vi "Hc2SequenceRunner.vi"() -> ()   [LabVIEW 2019]
uses:
  Components/DeltaRamp_globals.vi
  Components/B_Globals.vi
  Components/Global 2.vi
panel:
  in  "Set":bool
  in  "App":bool
  out "Settle Progress":u8(slide)=98 scale=0.0..100.0
  in  "Settle [Min]":dbl=1.0
  out "Numeric":i32=7
  in  "Base Name":string="RT_100uA"
  in  "Start":bool
  in  "Directory":path=path "C:/User Data/gy251/20210625 karine1B_Nb40-Dy20-Nb20-MgO2-Nb30/Out-of-plane"
  in  "T_high [K]":dbl=10.0
  in  "T_low [K]":dbl=2.0
  in  "dT/dt [K/min]":dbl=0.3
  in  "B_rate [T/min]":dbl=0.2
  in  "Set Fields, T_low, T_high":dbl[][](array[numeric])=[[0.0, 2.0, 10.0], [0.2, 2.0, 10.0], [0.4, 2.0, 10.0], [0.6, 2.0, 10.0], [0.8, 2.0, 10.0], [1.0, 2.0, 10.0], [1.5, 2.0, 10.0], [2.0, 2.0, 10.0], [2.5, 2.0, 10.0], [3.0, 2.0, 10.0], [3.5, 2.0, 10.0]]
  out "Action":string="Done/Wait for Start"
  out "Output File":path=path "RT_100uAapp=2p00T"
  # "Defaults"
  # "T_high -> Apply Field -> T_low"
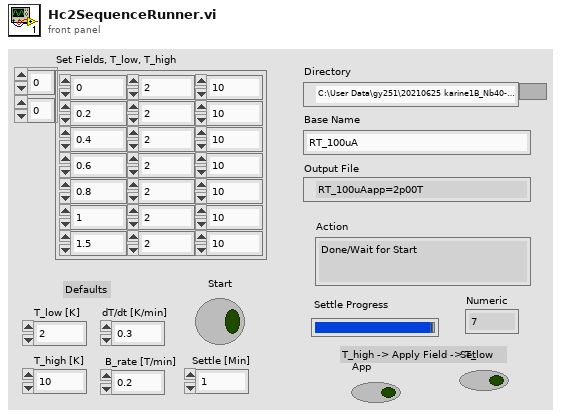
[diagram p1: front panel]
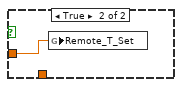
[diagram p3: hidden frame]
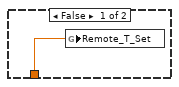
[diagram p4: hidden frame]
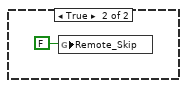
[diagram p5: hidden frame]
diagram:
  w2 = path ""
  n1 = global write "DeltaRamp_globals.vi" "Remote_Save_Directory"(w2) -> ()
  n2 = global write "DeltaRamp_globals.vi" "Remote_Ramp_Path"(w2) -> ()
  n3 = global write "DeltaRamp_globals.vi" "Remote_Save_String"("") -> ()
  n4 = while {
    stop <- FALSE stop-if-true
    n5 = local write "Action"("Done/Wait for Start") -> ()
    n6 = case shown="True" "Start" {
      frame False {
      }
      frame True {
        n7 = for {
          tunnel: "Set Fields, T_low, T_high" -> [w104] mode=indexing
          tunnel: "B_rate [T/min]" -> [w103]
          tunnel: "Directory" -> [w102]
          tunnel: "Base Name" -> [w101]
          tunnel: "T_low [K]" -> [w100]
          tunnel: "dT/dt [K/min]" -> [w99]
          tunnel: "T_high [K]" -> [w66]
          i -> [w98]
          n8 = flat-sequence {
            tunnel: w104 -> [w120]
            tunnel: w103 -> [w136]
            tunnel: w101 -> [w134]
            tunnel: [w127] -> w83
            tunnel: [w135] -> w81
            tunnel: w102 -> [w135]
            tunnel: [w122] -> w79
            tunnel: [w119] -> w77
            tunnel: w83 -> [w141]
            tunnel: [w141] -> w82
            tunnel: w81 -> [w140]
            tunnel: [w140] -> w80
            tunnel: w79 -> [w139]
            tunnel: [w139] -> w78
            tunnel: w77 -> [w138]
            tunnel: [w138] -> w76
            tunnel: [w143] -> w118
            tunnel: w82 -> [w143]
            tunnel: w80 -> [w142]
            tunnel: [w142] -> w117
            tunnel: w78 -> [w144]
            tunnel: w76 -> [w145]
            tunnel: [w145] -> w93
            tunnel: [w144] -> w88
            tunnel: w118 -> [w149]
            tunnel: [w149] -> w116
            tunnel: w117 -> [w148]
            tunnel: [w148] -> w115
            tunnel: [w147] -> w94
            tunnel: w93 -> [w147]
            tunnel: [w146] -> w89
            tunnel: w88 -> [w146]
            tunnel: [w153] -> w114
            tunnel: w116 -> [w153]
            tunnel: [w152] -> w113
            tunnel: w115 -> [w152]
            tunnel: [w151] -> w95
            tunnel: w94 -> [w151]
            tunnel: [w150] -> w90
            tunnel: w89 -> [w150]
            tunnel: [w162] -> w65
            tunnel: w114 -> [w162]
            tunnel: [w161] -> w63
            tunnel: w113 -> [w161]
            tunnel: [w160] -> w61
            tunnel: w95 -> [w160]
            tunnel: [w157] -> w59
            tunnel: w90 -> [w157]
            tunnel: w66 -> [w159]
            tunnel: w65 -> [w169]
            tunnel: [w169] -> w64
            tunnel: w63 -> [w168]
            tunnel: [w168] -> w62
            tunnel: w61 -> [w167]
            tunnel: [w167] -> w60
            tunnel: w59 -> [w166]
            tunnel: [w166] -> w58
            tunnel: [w174] -> w57
            tunnel: w64 -> [w174]
            tunnel: [w173] -> w55
            tunnel: w62 -> [w173]
            tunnel: [w172] -> w53
            tunnel: w60 -> [w172]
            tunnel: [w171] -> w51
            tunnel: w58 -> [w171]
            tunnel: w57 -> [w178]
            tunnel: [w178] -> w56
            tunnel: w55 -> [w177]
            tunnel: [w177] -> w54
            tunnel: w53 -> [w176]
            tunnel: [w176] -> w52
            tunnel: w51 -> [w175]
            tunnel: [w175] -> w50
            tunnel: [w184] -> w112
            tunnel: w56 -> [w184]
            tunnel: [w183] -> w111
            tunnel: w54 -> [w183]
            tunnel: [w182] -> w96
            tunnel: w52 -> [w182]
            tunnel: [w181] -> w91
            tunnel: w50 -> [w181]
            tunnel: w112 -> [w189]
            tunnel: w111 -> [w190]
            tunnel: [w190] -> w110
            tunnel: [w189] -> w109
            tunnel: [w188] -> w97
            tunnel: w96 -> [w188]
            tunnel: [w187] -> w92
            tunnel: w91 -> [w187]
            tunnel: [w198] -> w43
            tunnel: w110 -> [w198]
            tunnel: [w197] -> w41
            tunnel: w109 -> [w197]
            tunnel: [w196] -> w39
            tunnel: w97 -> [w196]
            tunnel: [w195] -> w37
            tunnel: w92 -> [w195]
            tunnel: w43 -> [w209]
            tunnel: [w209] -> w42
            tunnel: w41 -> [w207]
            tunnel: [w207] -> w40
            tunnel: w39 -> [w214]
            tunnel: [w214] -> w38
            tunnel: w37 -> [w213]
            tunnel: [w213] -> w36
            tunnel: [w218] -> w108
            tunnel: w42 -> [w218]
            tunnel: [w217] -> w107
            tunnel: w40 -> [w217]
            tunnel: w38 -> [w216]
            tunnel: w36 -> [w215]
            tunnel: [w216] -> w87
            tunnel: [w215] -> w84
            tunnel: w100 -> [w224]
            tunnel: w108 -> [w223]
            tunnel: w107 -> [w228]
            tunnel: [w228] -> w49
            tunnel: w99 -> [w221]
            tunnel: w87 -> [w222]
            tunnel: [w227] -> w47
            tunnel: w84 -> [w227]
            tunnel: [w223] -> w45
            tunnel: [w222] -> w30
            tunnel: [w221] -> w24
            tunnel: w49 -> [w237]
            tunnel: [w237] -> w48
            tunnel: w47 -> [w236]
            tunnel: [w236] -> w46
            tunnel: w45 -> [w235]
            tunnel: [w235] -> w44
            tunnel: [w233] -> w31
            tunnel: w30 -> [w233]
            tunnel: [w232] -> w25
            tunnel: w24 -> [w232]
            tunnel: [w242] -> w106
            tunnel: w48 -> [w242]
            tunnel: [w241] -> w85
            tunnel: w46 -> [w241]
            tunnel: [w240] -> w74
            tunnel: w44 -> [w240]
            tunnel: [w239] -> w32
            tunnel: w31 -> [w239]
            tunnel: [w238] -> w26
            tunnel: w25 -> [w238]
            tunnel: w106 -> [w249]
            tunnel: [w249] -> w105
            tunnel: [w248] -> w86
            tunnel: w85 -> [w248]
            tunnel: [w247] -> w75
            tunnel: w74 -> [w247]
            tunnel: [w246] -> w67
            tunnel: [w245] -> w33
            tunnel: w32 -> [w245]
            tunnel: [w244] -> w27
            tunnel: w26 -> [w244]
            tunnel: w105 -> [w259]
            tunnel: [w259] -> w73
            tunnel: w86 -> [w258]
            tunnel: [w258] -> w71
            tunnel: [w257] -> w69
            tunnel: w75 -> [w257]
            tunnel: w67 -> [w256]
            tunnel: [w255] -> w34
            tunnel: w33 -> [w255]
            tunnel: [w254] -> w28
            tunnel: w27 -> [w254]
            tunnel: w73 -> [w267]
            tunnel: [w267] -> w72
            tunnel: w71 -> [w266]
            tunnel: [w266] -> w70
            tunnel: w69 -> [w265]
            tunnel: [w265] -> w68
            tunnel: [w263] -> w35
            tunnel: w34 -> [w263]
            tunnel: [w262] -> w29
            tunnel: w28 -> [w262]
            tunnel: w72 -> [w269]
            tunnel: [w272] -> w23
            tunnel: w70 -> [w272]
            tunnel: w68 -> [w268]
            tunnel: w35 -> [w271]
            tunnel: w29 -> [w270]
            tunnel: [w271] -> w21
            tunnel: [w270] -> w19
            tunnel: [w269] -> w17
            tunnel: [w268] -> w15
            tunnel: w23 -> [w278]
            tunnel: [w278] -> w22
            tunnel: w21 -> [w277]
            tunnel: [w277] -> w20
            tunnel: w19 -> [w276]
            tunnel: [w276] -> w18
            tunnel: w17 -> [w275]
            tunnel: [w275] -> w16
            tunnel: w15 -> [w274]
            tunnel: [w274] -> w14
            tunnel: w22 -> [w281]
            tunnel: w66 -> [_]
            tunnel: w20 -> [w280]
            tunnel: w18 -> [w279]
            tunnel: w16 -> [w283]
            tunnel: w14 -> [w282]
            frame #0 {
              n9 = Index Array(array=w120, index=0) -> (element=w124:dbl)
              n10 = Number To Fractional String(number=w124, precision (6)=2) -> (F-format string=w132:string)  [unwired: 2 in]
              n11 = global write "B_Globals.vi" "Remote_set"(w124) -> ()
              n12 = global write "B_Globals.vi" "Remote_Rate"(w136) -> ()
              n13 = Index Array(array=w120, index=2) -> (element=w122:dbl)
              n14 = Index Array(array=w120, index=1) -> (element=w119:dbl)
              n15 = Search and Replace String(input string=w132, search string=".", replace string="p") -> (result string=w129:string)  [unwired: 5 in, 3 out]
              n16 = Concatenate Strings(w134, "app=", w129, "T") -> (w127:string)
            }
            frame #1 {
              w137 = TRUE
              n17 = global write "B_Globals.vi" "Remote_run"(w137) -> ()
              n18 = global write "B_Globals.vi" "Remote_Go"(w137) -> ()
            }
            frame #2 {
              # "Prep First File"
            }
            frame #3 {
            }
            frame #4 {
              n19 = local write "Action"("Waiting for B stable") -> ()
            }
            frame #5 {
              # "T_low"
              # "T_high"
              n20 = Not Equal?(x=0, y=w157) -> (x != y?=w155:bool)
              n21 = case shown="False" w155 {
                tunnel: w157 -> [_ w164]
                tunnel: w159 -> [w163 _]
                frame False {
                  n22 = global write "Global 2.vi" "Remote_T_Set"(w163) -> ()
                }
                frame True {
                  n23 = global write "Global 2.vi" "Remote_T_Set"(w164) -> ()
                }
              }
              n24 = global write "Global 2.vi" "Remote_T_Rate"(0.5) -> ()
            }
            frame #6 {
              n25 = global write "Global 2.vi" "Remote_T_GoTo"(TRUE) -> ()
            }
            frame #7 {
              n26 = Wait (ms)(milliseconds to wait=20000) -> ()  [unwired: 1 out]
            }
            frame #8 {
              n27 = while {
                stop <- w180 stop-if-true
                n28 = global read "Global 2.vi" "Sample_Stab"() -> (w180:bool)
                n29 = Wait (ms)(milliseconds to wait=500) -> ()  [unwired: 1 out]
              }
            }
            frame #9 {
              n30 = while {
                stop <- w185 stop-if-true
                n31 = global read "B_Globals.vi" "Rem_stable_B"() -> (w185:bool)
                n32 = Wait (ms)(milliseconds to wait=500) -> ()  [unwired: 1 out]
              }
            }
            frame #10 {
              n33 = global write "B_Globals.vi" "Remote_run"(FALSE) -> ()
            }
            frame #11 {
              n34 = Multiply(x="Settle [Min]", y=60) -> (x*y=w192:dbl)
              n35 = for {
                N: w192 -> [w200]
                i -> [w199]
                w206 = 1000
                n36 = Multiply(x=w206, y=w199) -> (x*y=w204:i32)
                n37 = Multiply(x=w206, y=w200) -> (x*y=w205:i32)
                n38 = Wait (ms)(milliseconds to wait=w206) -> ()  [unwired: 1 out]
                n39 = Divide(x=w204, y=w205) -> (x/y=w202:dbl)
                n40 = Multiply(x=100, y=w202) -> (x*y=→"Settle Progress":dbl)
              }
            }
            frame #12 {
              n41 = global write "DeltaRamp_globals.vi" "Remote_Save_Directory"(w209) -> ()
              n42 = Concatenate Strings(w207, "_cool.txt") -> (w211:string)
              n43 = Build Path(base path=w209, name or relative path=w211) -> (appended path=w210:path)
              n44 = String To Path(string=w207) -> (path=w208:path)
              n45 = global write "DeltaRamp_globals.vi" "Remote_Ramp_Path"(w210) -> ()
              n46 = local write "Output File"(w208) -> ()
              n47 = global write "DeltaRamp_globals.vi" "Remote_Save_String"(w211) -> ()
            }
            frame #13 {
              w220 = TRUE
              n48 = global write "DeltaRamp_globals.vi" "Remote_Measure"(w220) -> ()
              n49 = local write "Action"("Starting Measurement") -> ()
              n50 = global write "DeltaRamp_globals.vi" "Remote_Reset"(w220) -> ()
            }
            frame #14 {
              n51 = global write "Global 2.vi" "Remote_T_Rate"(w221) -> ()
              n52 = Not Equal?(x=0, y=w222) -> (x != y?=w226:bool)
              n53 = global write "Global 2.vi" "Remote_T_Ramp"(FALSE) -> ()
              n54 = case shown="True" w226 {
                tunnel: w222 -> [_ w231]
                tunnel: w224 -> [w230 _]
                frame False {
                  n55 = global write "Global 2.vi" "Remote_T_Set"(w230) -> ()
                }
                frame True {
                  n56 = global write "Global 2.vi" "Remote_T_Set"(w231) -> ()
                }
              }
            }
            frame #15 {
              w234 = TRUE
              n57 = global write "Global 2.vi" "Remote_T_Run"(w234) -> ()
              n58 = global write "Global 2.vi" "Remote_T_GoTo"(w234) -> ()
            }
            frame #16 {
              n59 = Wait (ms)(milliseconds to wait=20000) -> ()  [unwired: 1 out]
            }
            frame #17 {
              n60 = while {
                tunnel: [w250] -> w246
                stop <- w251 stop-if-true
                n61 = global read "Global 2.vi" "Sample_Stab"() -> (w252:bool)
                n62 = Wait (ms)(milliseconds to wait=500) -> ()  [unwired: 1 out]
                n63 = global read "DeltaRamp_globals.vi" "Remote_Skip"() -> (w250:bool)
                n64 = Or(x=w250, y=w252) -> (x .or. y?=w251:bool)
              }
            }
            frame #18 {
              n65 = case shown="False" w256 {
                frame False {
                  n66 = global write "DeltaRamp_globals.vi" "Remote_Ramp_Save"(TRUE) -> ()
                }
                frame True {
                  n67 = global write "DeltaRamp_globals.vi" "Remote_Skip"(FALSE) -> ()
                }
              }
            }
            frame #19 {
              n68 = Wait (ms)(milliseconds to wait=1000) -> ()  [unwired: 1 out]
            }
            frame #20 {
            }
            frame #21 {
              n69 = Wait (ms)(milliseconds to wait=1000) -> ()  [unwired: 1 out]
            }
            frame #22 {
              n70 = case shown="True" "Set" {
                tunnel: w280 -> [_ w291]
                tunnel: w279 -> [_ w290]
                tunnel: w283 -> [_ w288]
                tunnel: w282 -> [_ w289]
                tunnel: w281 -> [_ _]
                tunnel: w281 -> [_ w287]
                tunnel: w280 -> [_ w286]
                tunnel: w279 -> [_ w285]
                frame False {
                }
                frame True {
                  n71 = flat-sequence {
                    tunnel: w291 -> [_]
                    tunnel: w290 -> [_]
                    tunnel: w287 -> [w297]
                    tunnel: w289 -> [w304]
                    tunnel: w288 -> [w305]
                    tunnel: w286 -> [w310]
                    tunnel: w285 -> [w309]
                    frame #0 {
                      n72 = global write "B_Globals.vi" "Remote_set"(0.0) -> ()
                    }
                    frame #1 {
                      n73 = Wait (ms)(milliseconds to wait=5000) -> ()  [unwired: 1 out]
                    }
                    frame #2 {
                      n74 = while {
                        stop <- w294 stop-if-true
                        n75 = global read "B_Globals.vi" "Rem_stable_B"() -> (w294:bool)
                        n76 = Wait (ms)(milliseconds to wait=500) -> ()  [unwired: 1 out]
                      }
                    }
                    frame #3 {
                      n77 = global write "Global 2.vi" "Remote_T_Set"(w297) -> ()
                      n78 = global write "Global 2.vi" "Remote_T_Rate"(0.25) -> ()
                    }
                    frame #4 {
                      w298 = TRUE
                      n79 = global write "Global 2.vi" "Remote_T_Run"(w298) -> ()
                      n80 = global write "Global 2.vi" "Remote_T_GoTo"(w298) -> ()
                    }
                    frame #5 {
                      n81 = Wait (ms)(milliseconds to wait=10000) -> ()  [unwired: 1 out]
                    }
                    frame #6 {
                      n82 = while {
                        tunnel: [w300] -> _
                        stop <- w301 stop-if-true
                        n83 = global read "Global 2.vi" "Sample_Stab"() -> (w302:bool)
                        n84 = Wait (ms)(milliseconds to wait=500) -> ()  [unwired: 1 out]
                        n85 = global read "DeltaRamp_globals.vi" "Remote_Skip"() -> (w300:bool)
                        n86 = Or(x=w300, y=w302) -> (x .or. y?=w301:bool)
                      }
                    }
                    frame #7 {
                      n87 = global write "DeltaRamp_globals.vi" "Remote_Save_Directory"(w304) -> ()
                      n88 = Concatenate Strings(w305, "_set_cool.txt") -> (w307:string)
                      n89 = Build Path(base path=w304, name or relative path=w307) -> (appended path=w306:path)
                      n90 = global write "DeltaRamp_globals.vi" "Remote_Ramp_Path"(w306) -> ()
                      n91 = global write "DeltaRamp_globals.vi" "Remote_Save_String"(w307) -> ()
                    }
                    frame #8 {
                      w311 = TRUE
                      n92 = global write "Global 2.vi" "Remote_T_Rate"(w309) -> ()
                      n93 = global write "Global 2.vi" "Remote_T_Set"(w310) -> ()
                      n94 = global write "Global 2.vi" "Remote_T_Run"(w311) -> ()
                      n95 = global write "Global 2.vi" "Remote_T_GoTo"(w311) -> ()
                    }
                    frame #9 {
                      n96 = Wait (ms)(milliseconds to wait=5000) -> ()  [unwired: 1 out]
                    }
                    frame #10 {
                      n97 = while {
                        tunnel: [w313] -> _
                        stop <- w314 stop-if-true
                        n98 = global read "Global 2.vi" "Sample_Stab"() -> (w315:bool)
                        n99 = Wait (ms)(milliseconds to wait=500) -> ()  [unwired: 1 out]
                        n100 = global read "DeltaRamp_globals.vi" "Remote_Skip"() -> (w313:bool)
                        n101 = Or(x=w313, y=w315) -> (x .or. y?=w314:bool)
                      }
                    }
                    frame #11 {
                      n102 = global write "DeltaRamp_globals.vi" "Remote_Ramp_Save"(TRUE) -> ()
                    }
                  }
                }
              }
            }
            frame #23 {
            }
            frame #24 {
            }
            frame #25 {
            }
            frame #26 {
              n103 = global write "Global 2.vi" "Remote_T_Run"(FALSE) -> ()
              n104 = local write "Action"("Finished App Field Tc") -> ()
            }
          }
          "Numeric" <- w98
        }
        n105 = local write "Start"(FALSE) -> ()
      }
    }
  }
